vi "ReadFromOnlineDB.vi"(6 "Data format":enum16{"IDRA data", "XAM data"}(ring), 7 "SetLetto":bool=TRUE, 8 "error in":errorcluster, 10 "id_gara":i32=-1, 11 "Internet server":T5={"Web page telemetry"="http://telemetryh2polito.altervista.org/index.php/databaseio/getTelemetria", "Web page gps"="http://telemetryh2polito.altervista.org/index.php/databaseio/getGps"}) -> (0 "error out":errorcluster={"status"=TRUE, "code"=42, "source"="DataSocket Read in ReadFromOnlineDB.vi"}, 3 "Output packet":T3)   [LabVIEW 2015]
uses:
  Acquisition/Generic data packet.ctl
  My Graphs/Gps Map Graph coordinates.ctl
  Acquisition/IDRA Data Packet.ctl
  Acquisition/XAM Data Packet.ctl
  Acquisition/Acquisition.lvlib
panel:
  out "GpsResults":T1(array[cluster])
  out "TelemetriaResults":T2(array[cluster])
  out "GpsHtml":string
  out "TelemetriaHtml":string
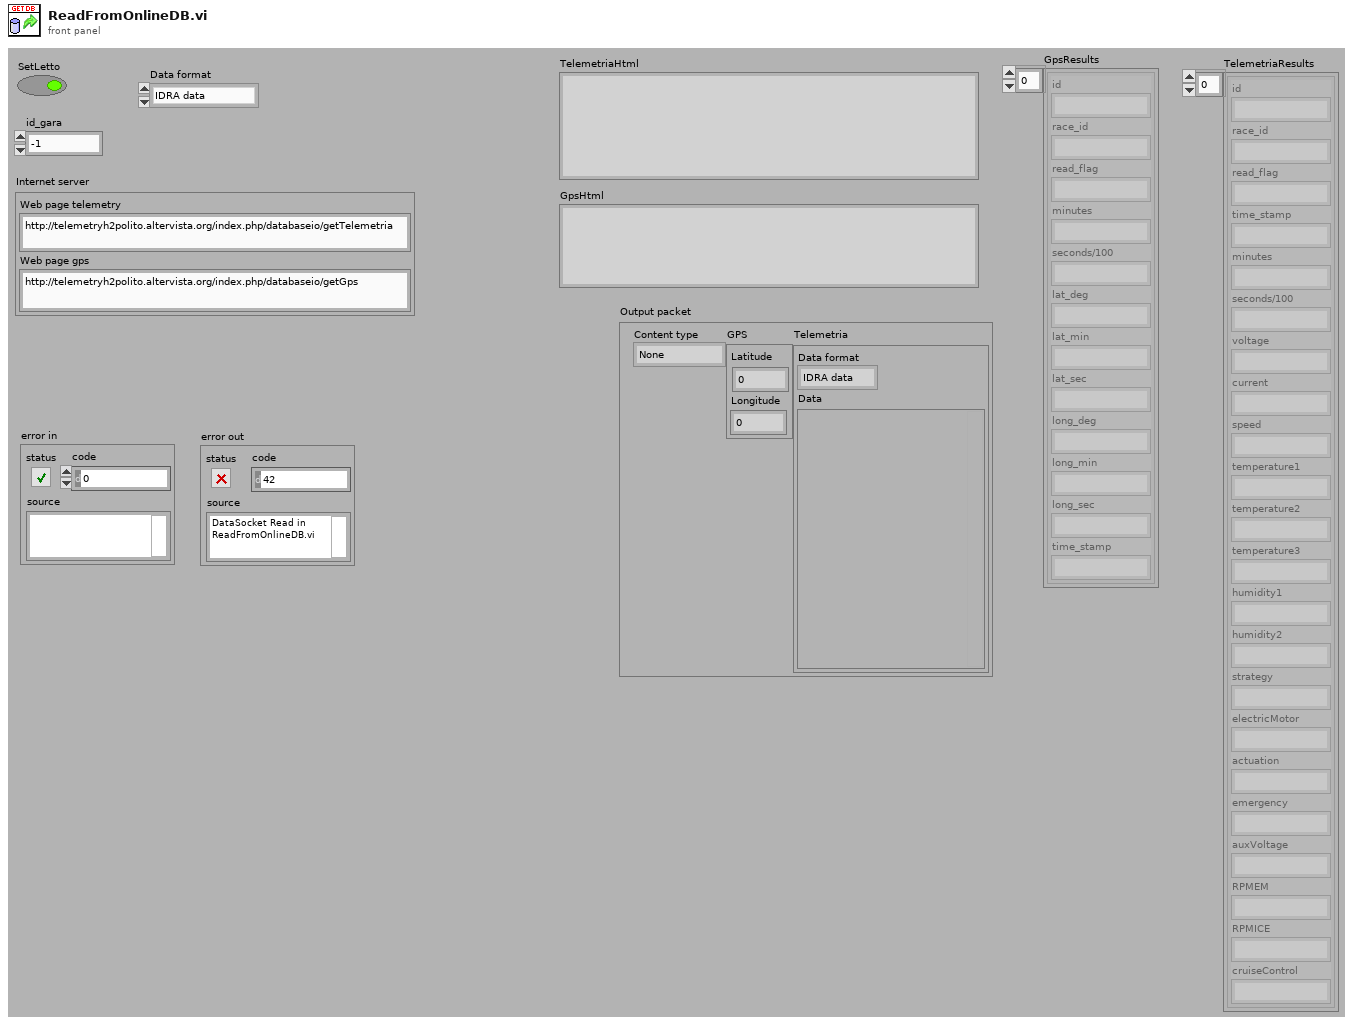
[diagram p1: front panel]
types:
  T1 = cluster{"id":string, "race_id":string, "read_flag":string, "minutes":string, "seconds/100":string, "lat_deg":string, "lat_min":string, "lat_sec":string, "long_deg":string, "long_min":string, "long_sec":string, "time_stamp":string}[]
  T2 = cluster{"id":string, "race_id":string, "read_flag":string, "time_stamp":string, "minutes":string, "seconds/100":string, "voltage":string, "current":string, "speed":string, "temperature1":string, "temperature2":string, "temperature3":string, "humidity1":string, "humidity2":string, "strategy":string, "electricMotor":string, "actuation":string, "emergency":string, "auxVoltage":string, "RPMEM":string, "RPMICE":string, "cruiseControl":string}[]
  T3 = typedef "Acquisition.lvlib/Generic data packet.ctl" = cluster{"Content type":enum16{"None", "Telemetria", "GPS"}, "GPS":T4, "Telemetria":cluster{"Data format":enum16{"IDRA data", "XAM data"}, "Data":variant}}
  T4 = typedef "Gps Map Graph coordinates.ctl" = cluster{"Latitude":dbl, "Longitude":dbl}
  T5 = cluster{"Web page telemetry":string, "Web page gps":string}
  T6 = cluster{"id":string, "race_id":string, "read_flag":string, "minutes":string, "seconds100":string, "lat_deg":string, "lat_min":string, "lat_sec":string, "long_deg":string, "long_min":string, "long_sec":string, "time_stamp":string}[]
  T7 = cluster{"id":string, "race_id":string, "read_flag":string, "time_stamp":string, "minutes":string, "seconds100":string, "voltage":string, "current":string, "speed":string, "temperature1":string, "temperature2":string, "temperature3":string, "humidity1":string, "humidity2":string, "strategy":string, "electricMotor":string, "actuation":string, "emergency":string, "auxVoltage":string, "RPMEM":string, "RPMICE":string, "cruiseControl":string}[]
  T8 = enum16{"Read", "Write", "ReadWrite", "BufferedRead", "BufferedReadWrite"}
  T9 = cluster{"Data format":enum16{"IDRA data", "XAM data"}, "Data":variant}
  T10 = typedef "Acquisition.lvlib/IDRA Data Packet.ctl" = cluster{"Minutes":u16, "Seconds/100":u16, "Voltage":sgl, "Current":sgl, "Speed":sgl, "Temperature 1":sgl, "Temperature 2":sgl, "Temperature 3":sgl, "Humidity 1":sgl, "Humidity 2":sgl, "Strategy":u8, "Electric Motor":bool, "Electronics":bool, "Emergency":bool}
  T11 = typedef "Acquisition.lvlib/XAM Data Packet.ctl" = cluster{"Minutes":u16, "Seconds/100":u16, "Supercap Voltage":sgl, "Battery Voltage":sgl, "Supercap Current":sgl, "Speed":sgl, "EM Temperature":sgl, "ECU Temperature":sgl, "ICE Temperature":sgl, "RPM EM":u16, "RPM ICE":u16, "Cruise Control":bool, "Emergency":bool}
  T12 = cluster{"id":string, "race_id":string, "read_flag":string, "minutes":string, "seconds100":string, "lat_deg":string, "lat_min":string, "lat_sec":string, "long_deg":string, "long_min":string, "long_sec":string, "time_stamp":string}
  T13 = cluster{"id":string, "race_id":string, "read_flag":string, "time_stamp":string, "minutes":string, "seconds100":string, "voltage":string, "current":string, "speed":string, "temperature1":string, "temperature2":string, "temperature3":string, "humidity1":string, "humidity2":string, "strategy":string, "electricMotor":string, "actuation":string, "emergency":string, "auxVoltage":string, "RPMEM":string, "RPMICE":string, "cruiseControl":string}
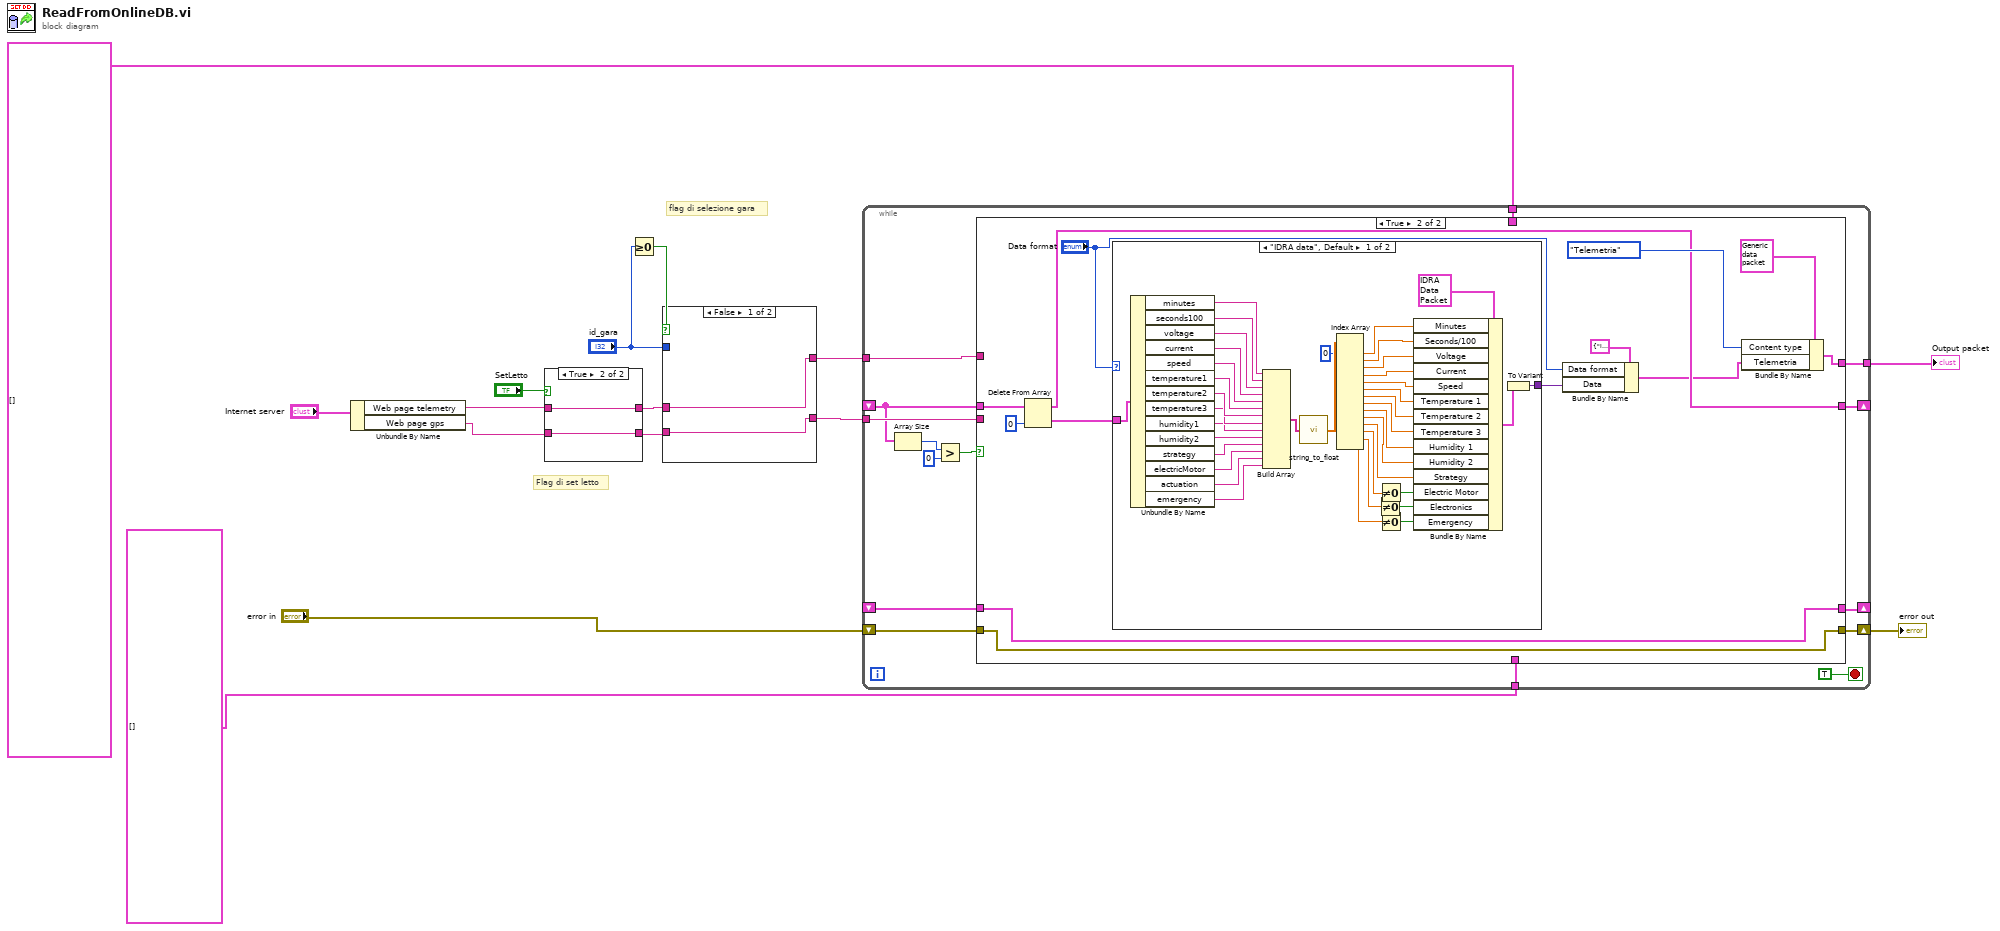
[diagram p0: block diagram]
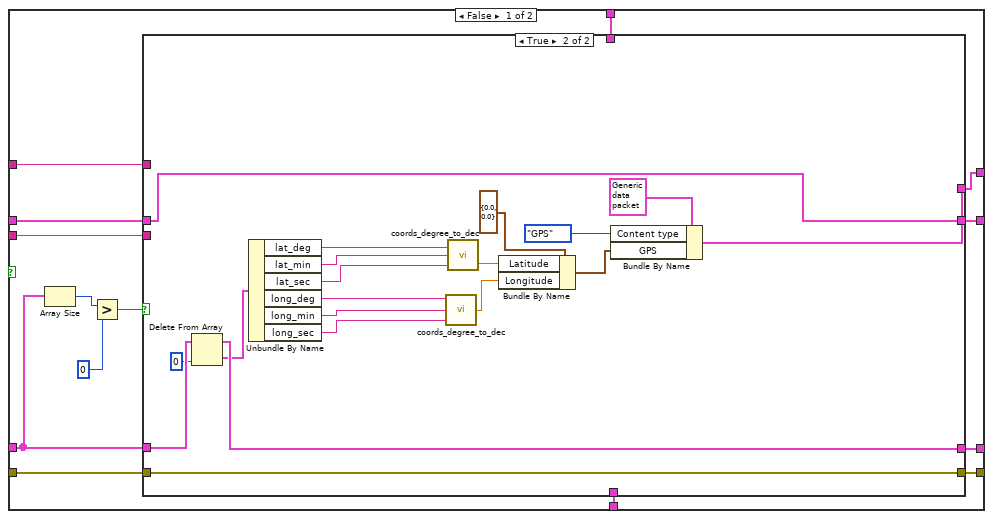
[diagram p2: hidden frame]
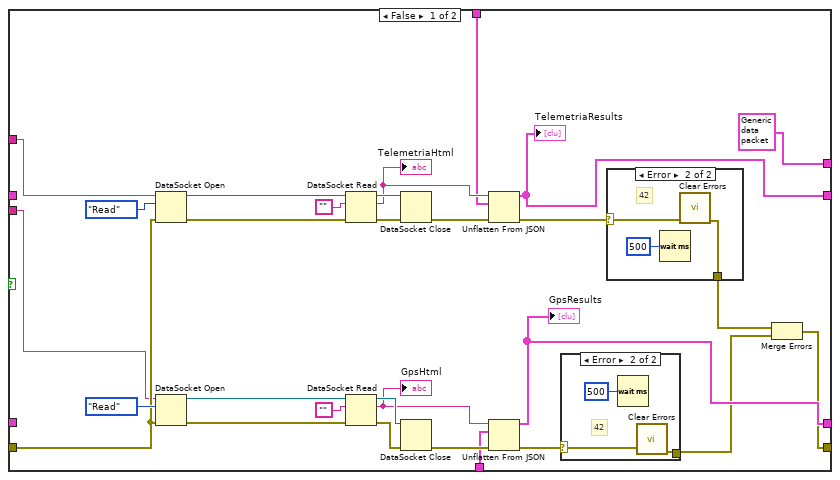
[diagram p3: hidden frame]
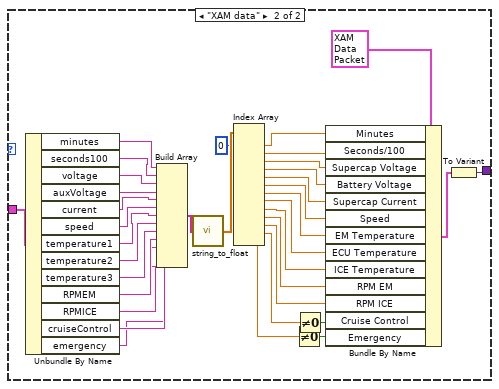
[diagram p6: hidden frame]
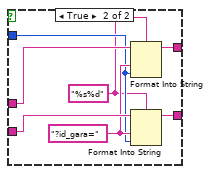
[diagram p7: hidden frame]
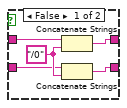
[diagram p8: hidden frame]
diagram:
  # "flag di selezione gara"
  # "Flag di set letto"
  n1 = Unbundle By Name("Internet server") -> ("Web page telemetry"=w6:string, "Web page gps"=w5:string)
  n2 = case shown="True" "SetLetto" {
    tunnel: w6 -> [w19 w22]
    tunnel: w5 -> [w18 w21]
    tunnel: [w17 w22] -> w13
    tunnel: [w16 w21] -> w12
    frame False {
      w20 = "/0"
      n3 = Concatenate Strings(w19, w20) -> (w17:string)
      n4 = Concatenate Strings(w18, w20) -> (w16:string)
    }
    frame True {
    }
  }
  n5 = Greater Or Equal To 0?(x="id_gara") -> (x >= 0?=w14:bool)
  n6 = case shown="False" w14 {
    tunnel: w13 -> [w24 w29]
    tunnel: [w24 w30] -> w9
    tunnel: w12 -> [w23 w28]
    tunnel: [w23 w31] -> w8
    tunnel: "id_gara" -> [_ w26]
    frame False {
    }
    frame True {
      w25 = "%s%d" ("format string")
      w27 = "?id_gara="
      n7 = Format Into String(format string=w25, initial string=w29, w27, w26) -> (resulting string=w30:string)  [unwired: 1 in, 1 out]
      n8 = Format Into String(format string=w25, initial string=w28, w27, w26) -> (resulting string=w31:string)  [unwired: 1 in, 1 out]
    }
  }
  n9 = while {
    tunnel: w9 -> [w45]
    tunnel: w8 -> [w44]
    shift-right: [w43] -> w3
    shift-left: "error in" -> [w46]
    shift-right: [w41] -> _
    shift-left: _ -> [w38]
    shift-right: [w40] -> _
    shift-left: _ -> [w39]
    tunnel: [w34] -> w4
    tunnel: T7 [] -> [w33]
    tunnel: T6 [] -> [w32]
    stop <- TRUE stop-if-true
    n10 = Array Size(array=w38) -> (size(s)=w37:i32)
    n11 = Greater?(x=w37, y=0) -> (0:w35:bool)
    n12 = case shown="True" w35 {
      tunnel: w46 -> [w60 w118]
      tunnel: w45 -> [w59 _]
      tunnel: w44 -> [w58 _]
      tunnel: [w57 w118] -> w43
      tunnel: [w56 w124] -> w41
      tunnel: [w55 w117] -> w40
      tunnel: w38 -> [w50 w125]
      tunnel: w39 -> [w51 w117]
      tunnel: [w49 w128] -> w34
      tunnel: w33 -> [w48 _]
      tunnel: w32 -> [w47 _]
      frame False {
        n13 = Array Size(array=w51) -> (size(s)=w53:i32)
        n14 = Greater?(x=w53, y=0) -> (0:w52:bool)
        n15 = case shown="True" w52 {
          tunnel: w60 -> [w73 w109]
          tunnel: w59 -> [w72 _]
          tunnel: w58 -> [w71 _]
          tunnel: [w64 w109] -> w57
          tunnel: [w70 w111] -> w56
          tunnel: [w69 w112] -> w55
          tunnel: w51 -> [_ w114]
          tunnel: w50 -> [_ w111]
          tunnel: [T3 {"Content type"=enum."None", "GPS"={"Latitude"=0.0, "Longitude"=0.0}, "Telemetria"={"Data format"=enum."IDRA data", "Data"=variant}} w108] -> w49
          tunnel: w48 -> [w62 _]
          tunnel: w47 -> [w61 _]
          frame False {
            n16 = DataSocket Open(8:w73, 10:T8."Read" ("mode"), 11:w72) -> (0:w86:errorcluster, 3:w89:refnum<k13>)  [unwired: 1 in]
            n17 = DataSocket Open(8:w73, 10:T8."Read" ("mode"), 11:w71) -> (0:w78:errorcluster, 3:w81:refnum<k13>)  [unwired: 1 in]
            n18 = DataSocket Read(8:w86, 10:"", 11:w89) -> (0:w87:errorcluster, 2:w84:string, 3:w88:refnum<k13>)  [unwired: 2 in, 4 out]
            "TelemetriaHtml" <- w84
            n19 = DataSocket Read(8:w78, 10:"", 11:w81) -> (0:w79:errorcluster, 2:w76:string, 3:w80:refnum<k13>)  [unwired: 2 in, 4 out]
            "GpsHtml" <- w76
            n20 = DataSocket Close(8:w87, 11:w88) -> (0:w83:errorcluster)  [unwired: 1 in, 1 out]
            n21 = DataSocket Close(8:w79, 11:w80) -> (0:w75:errorcluster)  [unwired: 1 in, 1 out]
            n22 = Unflatten From JSON(JSON string=w84, type and defaults=w62, error in (no error)=w83) -> (value=w70:T7, error out=w66:errorcluster)  [unwired: 4 in]
            "TelemetriaResults" <- w70
            n23 = Unflatten From JSON(JSON string=w76, type and defaults=w61, error in (no error)=w75) -> (value=w69:T6, error out=w65:errorcluster)  [unwired: 4 in]
            "GpsResults" <- w69
            n24 = case shown="Error" w65 {
              selector: w65 -> [w90 w92]
              tunnel: [w90 w93] -> w67
              frame No Error {
              }
              frame Error {
                # "42"
                n25 = Wait (ms)(milliseconds to wait=u32 500) -> ()  [unwired: 1 out]
                n26 = call <vilib>:"Clear Errors.vi"("error in (no error)"=w92) -> ("error out"=w93:errorcluster)  [unwired: 5 in, 1 out]
              }
            }
            n27 = case shown="Error" w66 {
              selector: w66 -> [w94 w96]
              tunnel: [w94 w97] -> w68
              frame No Error {
              }
              frame Error {
                # "42"
                n28 = Wait (ms)(milliseconds to wait=u32 500) -> ()  [unwired: 1 out]
                n29 = call <vilib>:"Clear Errors.vi"("error in (no error)"=w96) -> ("error out"=w97:errorcluster)  [unwired: 5 in, 1 out]
              }
            }
            n30 = Merge Errors(w68, w67) -> (w64:errorcluster)
          }
          frame True {
            n31 = Delete From Array(array=w114, index=0) -> (deleted portion=w110:T12, array with subset deleted=w112:T6)  [unwired: 1 in]
            n32 = Unbundle By Name(w110) -> ("lat_deg"=w103:string, "lat_min"=w102:string, "lat_sec"=w101:string, "long_deg"=w100:string, "long_min"=w99:string, "long_sec"=w98:string)
            n33 = call "coords_degree_to_dec.vi"("Seconds"=w98, "Minutes"=w99, "Degrees"=w100) -> ("Decimal"=w104:dbl)
            n34 = call "coords_degree_to_dec.vi"("Seconds"=w101, "Minutes"=w102, "Degrees"=w103) -> ("Decimal"=w105:dbl)
            n35 = Bundle By Name(cluster=T4 {"Latitude"=0.0, "Longitude"=0.0} ("GPS"), "Latitude"=w105, "Longitude"=w104) -> (w107:T4)
            n36 = Bundle By Name(cluster=T3 {"Content type"=enum."None", "GPS"={"Latitude"=0.0, "Longitude"=0.0}, "Telemetria"={"Data format"=enum."IDRA data", "Data"=variant}}, "Content type"=enum16{"None", "Telemetria", "GPS"}."GPS", "GPS"=w107) -> (w108:T3)
          }
        }
      }
      frame True {
        n37 = Delete From Array(array=w125, index=0) -> (deleted portion=w120:T13, array with subset deleted=w124:T7)  [unwired: 1 in]
        n38 = case shown="\"IDRA data\", Default" "Data format" {
          tunnel: [w166 w200] -> w121
          tunnel: w120 -> [w164 w199]
          frame "IDRA data", Default {
            n39 = Unbundle By Name(w164) -> ("minutes"=w163:string, "seconds100"=w162:string, "voltage"=w161:string, "current"=w160:string, "speed"=w159:string, "temperature1"=w158:string, "temperature2"=w157:string, "temperature3"=w156:string, "humidity1"=w155:string, "humidity2"=w154:string, "strategy"=w153:string, "electricMotor"=w152:string, "actuation"=w151:string, "emergency"=w150:string)
            n40 = Build Array(w163, w162, w161, w160, w159, w158, w157, w156, w155, w154, w153, w152, w151, w150) -> (w149:string[])
            n41 = call "string_to_float.vi"("Array in"=w149) -> ("Array out"=w148:dbl[])
            n42 = Index Array(array=w148, index #1=0 ("index")) -> (element #1=w146:dbl, element #2=w145:dbl, element #3=w144:dbl, element #4=w143:dbl, element #5=w142:dbl, element #6=w141:dbl, element #7=w140:dbl, element #8=w139:dbl, element #9=w138:dbl, element #10=w137:dbl, element #11=w136:dbl, element #12=w132:dbl, element #13=w131:dbl, element #14=w130:dbl)  [unwired: 13 in]
            n43 = Not Equal To 0?(x=w131) -> (x != 0?=w134:bool)
            n44 = Not Equal To 0?(x=w132) -> (x != 0?=w135:bool)
            n45 = Not Equal To 0?(x=w130) -> (x != 0?=w133:bool)
            n46 = Bundle By Name(cluster=T10 {"Minutes"=0, "Seconds/100"=0, "Voltage"=0.0, "Current"=0.0, "Speed"=0.0, "Temperature 1"=0.0, "Temperature 2"=0.0, "Temperature 3"=0.0, "Humidity 1"=0.0, "Humidity 2"=0.0, "Strategy"=0, "Electric Motor"=FALSE, "Electronics"=FALSE, "Emergency"=FALSE} ("IDRA Data Packet"), "Minutes"=w146, "Seconds/100"=w145, "Voltage"=w144, "Current"=w143, "Speed"=w142, "Temperature 1"=w141, "Temperature 2"=w140, "Temperature 3"=w139, "Humidity 1"=w138, "Humidity 2"=w137, "Strategy"=w136, "Electric Motor"=w135, "Electronics"=w134, "Emergency"=w133) -> (w165:T10)
            n47 = To Variant(anything=w165) -> (Variant=w166:variant)
          }
          frame "XAM data" {
            n48 = Unbundle By Name(w199) -> ("minutes"=w181:string, "seconds100"=w180:string, "voltage"=w179:string, "auxVoltage"=w178:string, "current"=w177:string, "speed"=w176:string, "temperature1"=w175:string, "temperature2"=w174:string, "temperature3"=w173:string, "RPMEM"=w172:string, "RPMICE"=w169:string, "cruiseControl"=w170:string, "emergency"=w168:string)
            n49 = Build Array(w181, w180, w179, w178, w177, w176, w175, w174, w173, w172, w169, w170, w168) -> (w171:string[])
            n50 = call "string_to_float.vi"("Array in"=w171) -> ("Array out"=w198:dbl[])
            n51 = Index Array(array=w198, index #1=0 ("index")) -> (element #1=w196:dbl, element #2=w195:dbl, element #3=w194:dbl, element #4=w193:dbl, element #5=w192:dbl, element #6=w191:dbl, element #7=w190:dbl, element #8=w189:dbl, element #9=w188:dbl, element #10=w187:dbl, element #11=w186:dbl, element #12=w183:dbl, element #13=w182:dbl)  [unwired: 12 in]
            n52 = Not Equal To 0?(x=w182) -> (x != 0?=w184:bool)
            n53 = Not Equal To 0?(x=w183) -> (x != 0?=w185:bool)
            n54 = Bundle By Name(cluster=T11 {"Minutes"=0, "Seconds/100"=0, "Supercap Voltage"=0.0, "Battery Voltage"=0.0, "Supercap Current"=0.0, "Speed"=0.0, "EM Temperature"=0.0, "ECU Temperature"=0.0, "ICE Temperature"=0.0, "RPM EM"=0, "RPM ICE"=0, "Cruise Control"=FALSE, "Emergency"=FALSE} ("XAM Data Packet"), "Minutes"=w196, "Seconds/100"=w195, "Supercap Voltage"=w194, "Battery Voltage"=w193, "Supercap Current"=w192, "Speed"=w191, "EM Temperature"=w190, "ECU Temperature"=w189, "ICE Temperature"=w188, "RPM EM"=w187, "RPM ICE"=w186, "Cruise Control"=w185, "Emergency"=w184) -> (w201:T11)
            n55 = To Variant(anything=w201) -> (Variant=w200:variant)
          }
        }
        n56 = Bundle By Name(cluster=T9 {"Data format"=enum."IDRA data", "Data"=variant} ("Telemetria"), "Data format"="Data format", "Data"=w121) -> (w119:T9)
        n57 = Bundle By Name(cluster=T3 {"Content type"=enum."None", "GPS"={"Latitude"=0.0, "Longitude"=0.0}, "Telemetria"={"Data format"=enum."IDRA data", "Data"=variant}}, "Content type"=enum16{"None", "Telemetria", "GPS"}."Telemetria", "Telemetria"=w119) -> (w128:T3)
      }
    }
  }
  "error out" <- w3
  "Output packet" <- w4
